vi "Write Slider Marker Values[].vi"(5 "Marker Values[]":dbl[](array[numeric]), 9 "SlideScale in":refnum<class "SlideScale.lvclass">) -> (3 "SlideScale out":refnum<class "SlideScale.lvclass">)   [LabVIEW 2014, in "SlideScale.lvclass"]
uses:
  SlideScale.lvclass
  SlideScale.lvclass/SlideScale.ctl
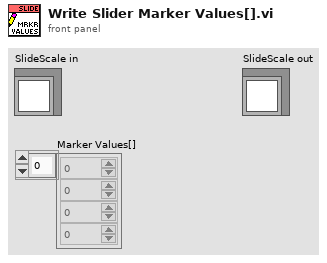
[diagram p1: front panel]
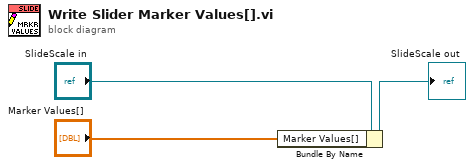
[diagram p0: block diagram]
diagram:
  n1 = Bundle By Name(cluster="SlideScale in", "Marker Values[]"="Marker Values[]") -> (→"SlideScale out":refnum<class "SlideScale.lvclass">)
